vi "Test web client.vi"() -> ()   [LabVIEW 2015]
uses:
  <vilib>/httpClient/LabVIEWHTTPClient.lvlib
panel:
  out "body":string
  out "headers":string
  in  "URL":string
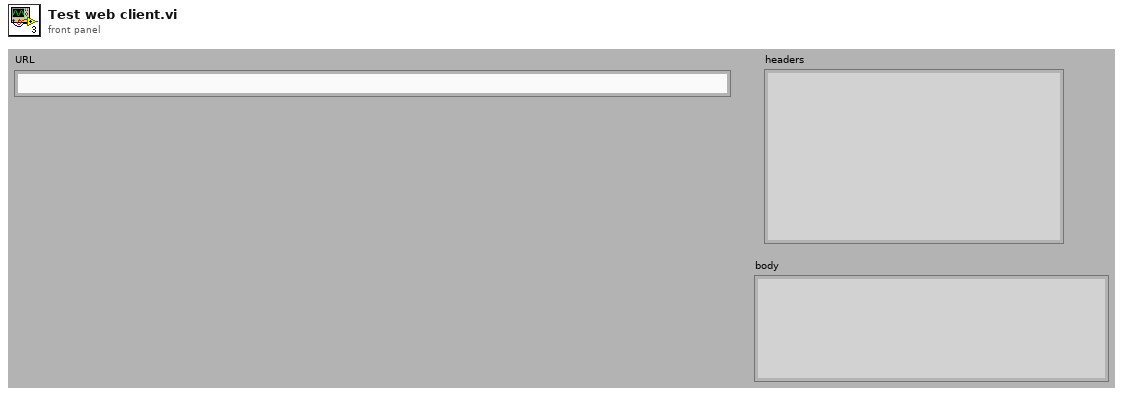
[diagram p1: front panel]
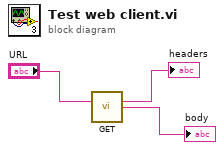
[diagram p0: block diagram]
diagram:
  n1 = call <vilib>:"GET.vi"("url"="URL") -> ("headers"=→"headers":string, "body"=→"body":string)  [unwired: 11 in, 2 out]
